vi "fftGetMags.vi"(6 "unit cal, scu":dbl=1000.0, 8 "660 F (Hz)":i32, 9 "532 F (Hz)":i32, 10 "405 F (Hz)":i32, 11 "input cluster":cluster{"f0":dbl, "df":dbl, "magnitude":dbl[]}) -> (0 "mag660 (mV)":dbl, 1 "mag532 (mV)":dbl, 2 "mag405 (mV)":dbl)   [LabVIEW 2011]
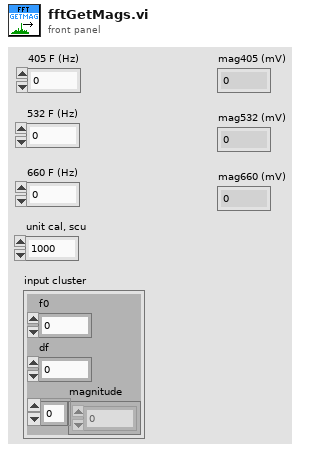
[diagram p1: front panel]
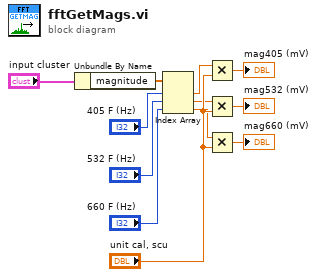
[diagram p0: block diagram]
diagram:
  n1 = Unbundle By Name("input cluster") -> ("magnitude"=w2:dbl[])
  n2 = Index Array(array=w2, index #1="405 F (Hz)", index #2="532 F (Hz)", index #3="660 F (Hz)") -> (element #1=w5:dbl, element #2=w3:dbl, element #3=w4:dbl)
  n3 = Multiply(x=w5, y="unit cal, scu") -> (x*y=→"mag405 (mV)":dbl)
  n4 = Multiply(x=w3, y="unit cal, scu") -> (x*y=→"mag532 (mV)":dbl)
  n5 = Multiply(x=w4, y="unit cal, scu") -> (x*y=→"mag660 (mV)":dbl)
